vi "ChangeStatusCmdCluster.vi"(9 "status":string, 11 "CmdClusterIN":T2) -> (3 "CmdClusterOUT":T1)   [LabVIEW 2011]
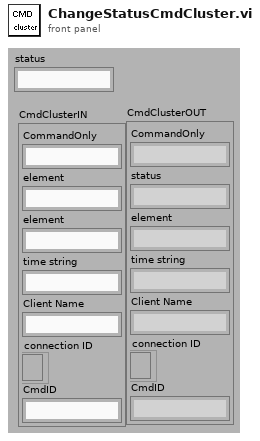
[diagram p1: front panel]
types:
  T1 = cluster{"CommandOnly":string, "status":string, "element":string, "time string":string, "Client Name":string, "connection ID":refnum<k5>, "CmdID":string}
  T2 = cluster{"CommandOnly":string, "element":string, "element":string, "time string":string, "Client Name":string, "connection ID":refnum<k5>, "CmdID":string}
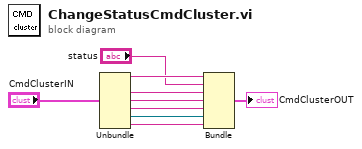
[diagram p0: block diagram]
diagram:
  n1 = Unbundle("CmdClusterIN") -> ("CommandOnly"=w8:string, "element"=w7:string, "time string"=w6:string, "Client Name"=w5:string, "connection ID"=w4:refnum<k5>, "CmdID"=w3:string)  [unwired: 1 out]
  n2 = Bundle("CommandOnly"=w8, "status"="status", "element"=w7, "time string"=w6, "Client Name"=w5, "connection ID"=w4, "CmdID"=w3) -> (→"CmdClusterOUT":T1)  [unwired: 1 out]
